vi "AutoPilot.vi"(3 "human contribution":dbl, 4 "State":bool) -> (0 "End Contribution":dbl)   [LabVIEW 2018]
uses:
  SensorReadings.vi
panel:
  in  "Plot PID":bool
  out "PID Tracking":cluster{"Goal Wheel Position":dbl, dbl}(graph)={"Goal Wheel Position"=0.0, -6.7188720703125}
  out "Contribution Tracking":cluster{dbl, dbl, dbl}(graph)={0.335943603515625, 0.10438529174803275, -0.0}
  in  "Autopilot Deadband (deg)":dbl=1.0
  in  "Kp Butterfly":dbl=0.05
  in  "Ki Butterfly":dbl=0.008
  in  "Kd Butterfly":dbl
  in  "N-Diff Butterfly":i32=50
  in  "N-Int Butterfly":i32=50
  in  "Kf Butterfly":dbl=0.5
  in  "Kp Traction":dbl=0.05
  in  "Ki Traction":dbl=0.008
  in  "Kd Traction":dbl
  in  "N-Diff Traction":i32=50
  in  "N-Int Traction":i32=50
  in  "Kf Traction":dbl=0.5
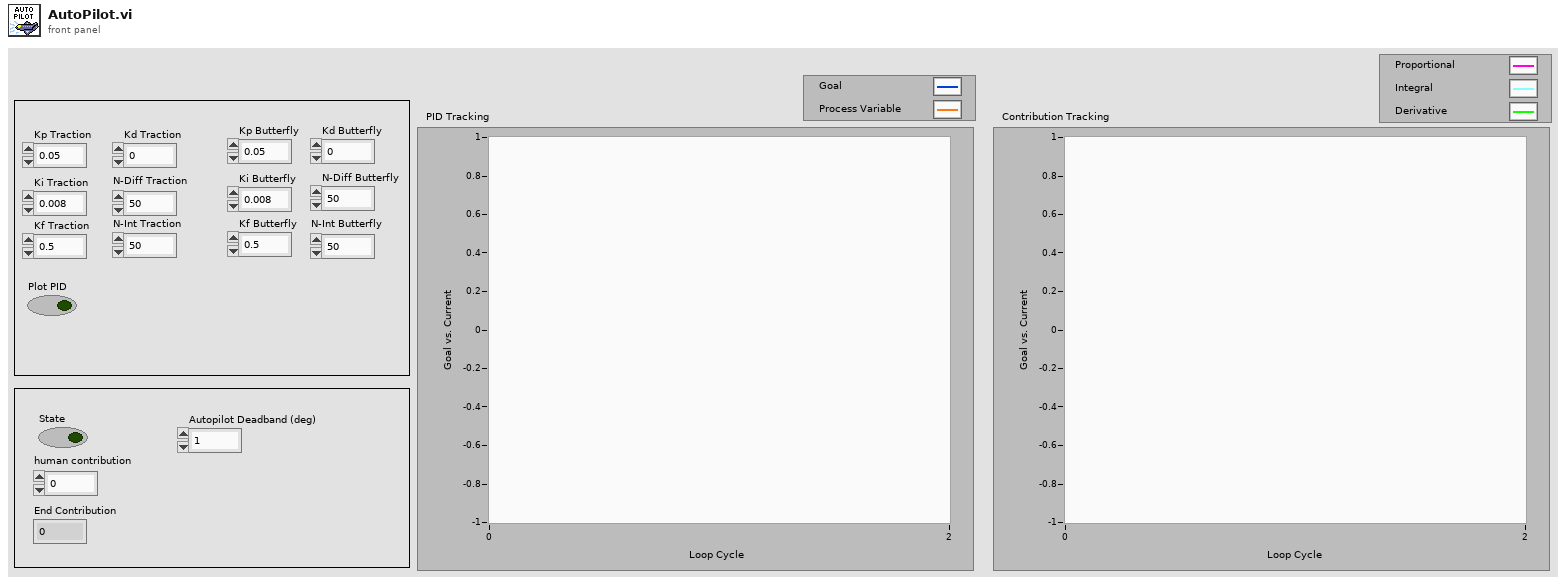
[diagram p1: front panel]
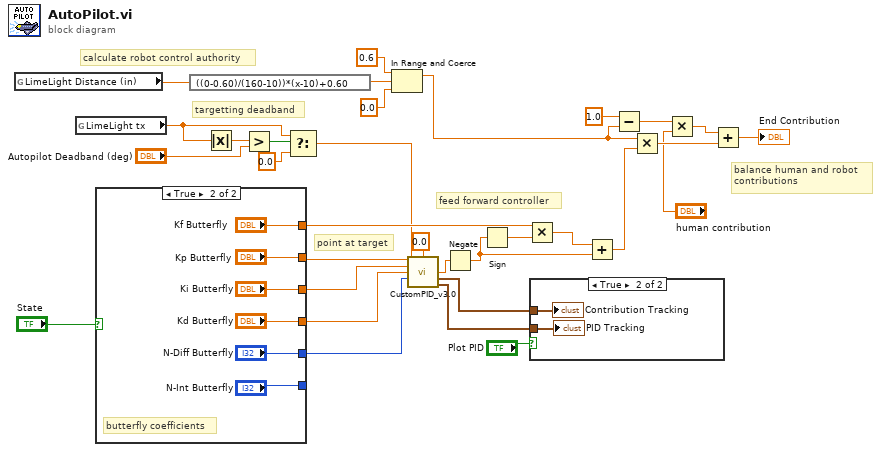
[diagram p0: block diagram]
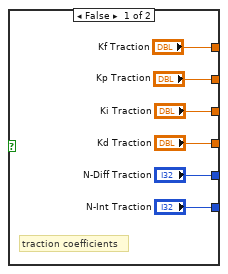
[diagram p3: hidden frame]
diagram:
  # "point at target"
  # "calculate robot control authority"
  # "balance human and robot\ncontributions"
  # "targetting deadband"
  # "feed forward controller"
  n1 = global read "SensorReadings.vi" "LimeLight Distance (in)"() -> (w23:dbl)
  n2 = global read "SensorReadings.vi" "LimeLight tx"() -> (w8:dbl)
  n3 = case shown="True" "State" {
    tunnel: ["Kp Traction" "Kp Butterfly"] -> w32
    tunnel: ["Ki Traction" "Ki Butterfly"] -> w31
    tunnel: ["Kd Traction" "Kd Butterfly"] -> w30
    tunnel: ["N-Diff Traction" "N-Diff Butterfly"] -> w29
    tunnel: ["N-Int Traction" "N-Int Butterfly"] -> _
    tunnel: ["Kf Traction" "Kf Butterfly"] -> w15
    frame False {
      # "traction coefficients"
    }
    frame True {
      # "butterfly coefficients"
    }
  }
  n4 = expression code="((0-0.60)/(160-10))*(x-10)+0.60"(w23) -> (w22:dbl)
  n5 = Absolute Value(x=w8) -> (abs(x)=w10:dbl)
  n6 = Greater?(x=w10, y="Autopilot Deadband (deg)") -> (0:w9:bool)
  n7 = Select(t=w8, s=w9, f=0.0) -> (s? t:f=w7:dbl)
  n8 = In Range and Coerce(upper limit=0.6, x=w22, lower limit=0.0) -> (coerced(x)=w19:dbl)  [unwired: 1 out]
  n9 = call "CustomPID_v3.0.vi"("Kp"=w32, "Process Variable"=w7, "Goal"=0.0, "Ki"=w31, "Kd"=w30, "N-Diff"=w29) -> ("Command"=w13:dbl, "Contribution Tracking"=w27:cluster{dbl, dbl, dbl}, "PID Tracking"=w28:cluster{"Goal Wheel Position":dbl, dbl})  [unwired: 6 in, 1 out]
  n10 = Negate(x=w13) -> (-x=w11:dbl)
  n11 = Sign(1:w11) -> (0:w12:dbl)
  n12 = Multiply(x=w15, y=w12) -> (x*y=w14:dbl)
  n13 = case shown="True" "Plot PID" {
    tunnel: w28 -> [_ w46]
    tunnel: w27 -> [_ w45]
    frame False {
    }
    frame True {
      "PID Tracking" <- w46
      "Contribution Tracking" <- w45
    }
  }
  n14 = Add(x=w14, y=w11) -> (x+y=w16:dbl)
  n15 = Subtract(x=1.0, y=w19) -> (x-y=w20:dbl)
  n16 = Multiply(x=w19, y=w16) -> (x*y=w24:dbl)
  n17 = Multiply(x=w20, y="human contribution") -> (x*y=w25:dbl)
  n18 = Add(x=w25, y=w24) -> (x+y=→"End Contribution":dbl)
